vi "Read Variant Key.vi"(5 "format string (%;%f)":string="%f", 7 "section":string, 8 "error in (no error)":errorcluster, 9 "type":variant, 10 "key (optional)":string, 11 "refnum":T1) -> (0 "error out":errorcluster, 1 "key-value":variant, 2 "found?":bool, 3 "refnum out":T1)   [LabVIEW 2017, in "INI++.lvlib"]
doc: "Reads a value associated with key in a specified section of the configuration data identified by refnum. If \"key\" input is not specified, the name of the variant object is used as the key. the \"found?\" output will be TRUE for compount objects (clusters) only if all elements (recursively) are found.\n\nFor example a Boolean named \"Enable\" with a value of TRUE would correspond to the key-value pair:\n\nEnable=TRUE\n\nNote: Special characters in section and key names will be escape-coded. These include the following: \\00-\\1F (non-printable chars); \"[\", \"]\", and \"=\" (INI syntax elements); \\FE (\"þ\") and \\FF (\"ÿ\") (legacy bracket encoding); Additionally, the escape character, \"\\\", will be escaped as \"\\\\\"."
uses:
  Candidate/INI/INI++.lvlib
  <vilib>/Utility/config.llb/NI_LVConfig.lvlib
  <vilib>/Utility/config.llb/Read Key (String).vi
  <vilib>/Utility/config.llb/Read Key (Double).vi
  <vilib>/Utility/Data Type/NI_Data Type.lvlib
  <vilib>/Utility/Data Type/Type Definitions/Data Type.ctl
  _openG/_reuse_openG.lvlib
  <vilib>/Utility/config.llb/Read Key (Boolean).vi
  <vilib>/Utility/config.llb/Read Key (Path).vi
  <vilib>/Utility/config.llb/Read Key (U32).vi
  <vilib>/Utility/config.llb/Read Key (I32).vi
  <vilib>/Utility/config.llb/Config Data RefNum.ctl
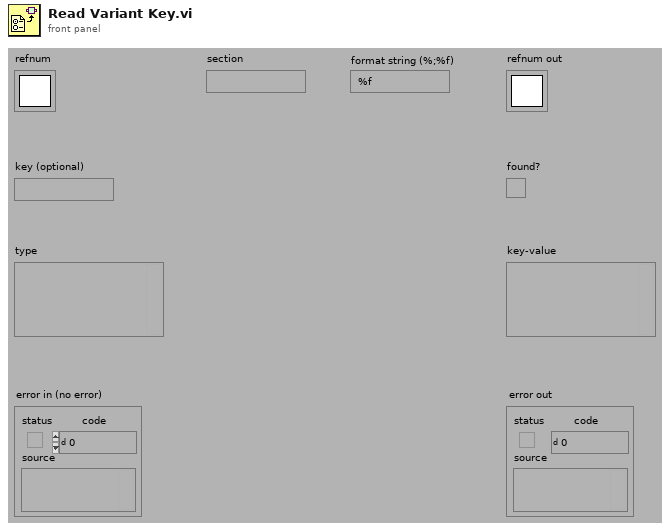
[diagram p1: front panel]
types:
  T1 = typedef "NI_LVConfig.lvlib/Config Data RefNum.ctl" = refnum<k1>
  T2 = typedef "NI_Data Type.lvlib/Data Type.ctl" = enum8{"Invalid Type", "Void", "I8", "I16", "I32", "I64", "U8", "U16", "U32", "U64", "Single Float", "Double Float", "Extended Float", "Single Complex", "Double Complex", "Extended Complex", "Enum U8", "Enum U16", "Enum U32", "Enum U64", "Single Float With Unit", "Double Float With Unit", "Extended Float With Unit", "Single Complex with Unit", "Double Complex with Unit", "Extended Complex with Unit", "Boolean", "String", "Path", "Picture", "Tag", "Array", "Cluster", "Variant", "LV Variant", "Waveform", "Timestamp", "Digital Waveform", "Digital Data", "ExpressData", "Refnum", "External Data", "VI", "Poly VI", "LabVIEW Class Instance", "Fixed Point"}
  T3 = typedef "Type Descriptor__ogtk.ctl" = i16[]
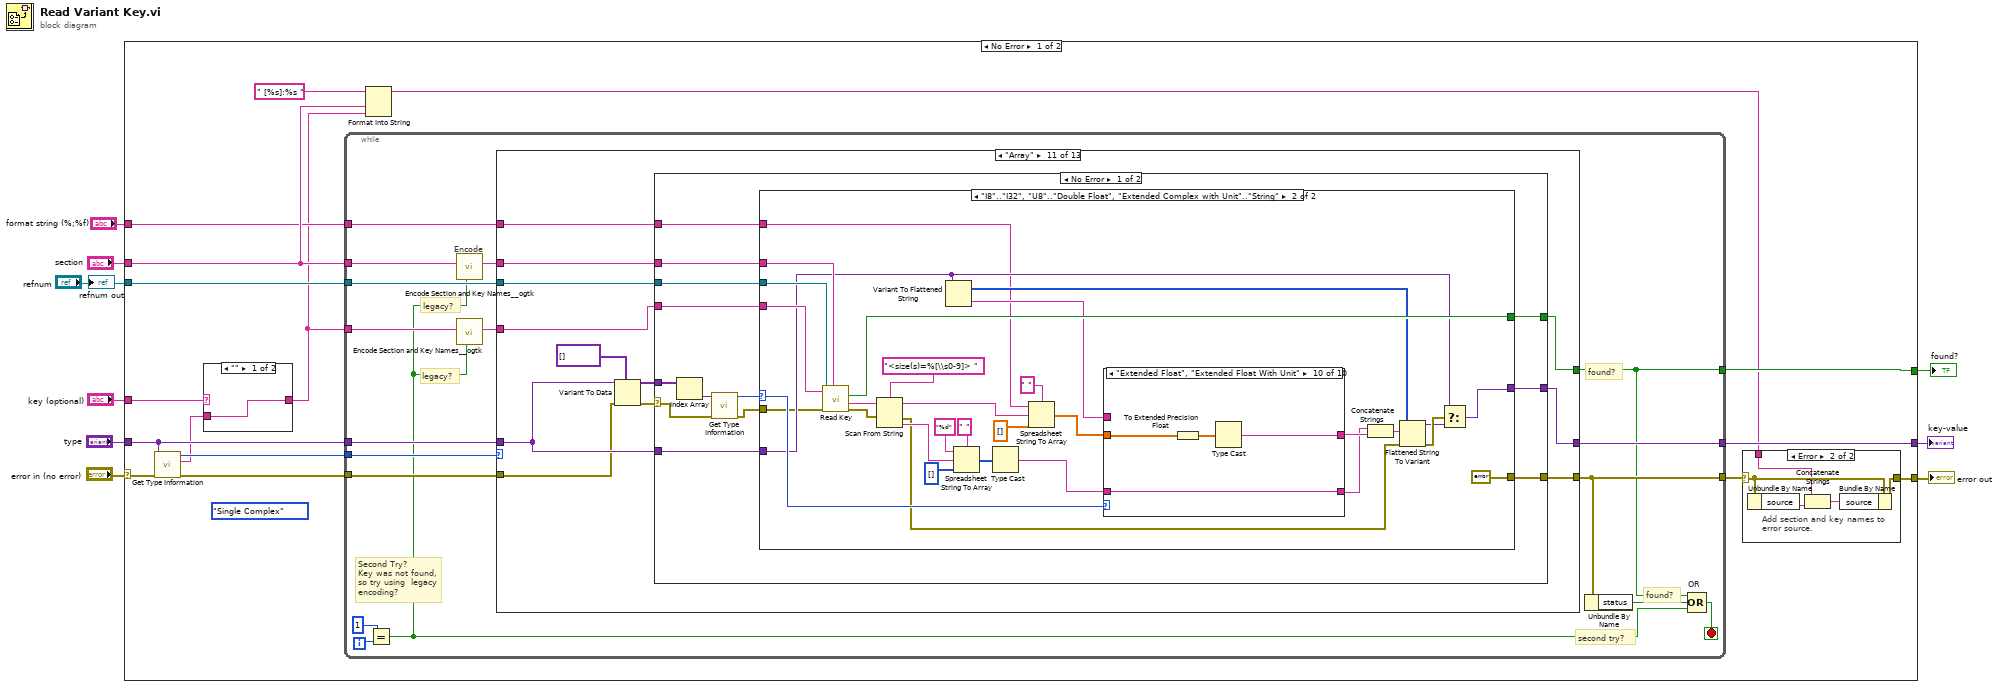
[diagram p0: block diagram]
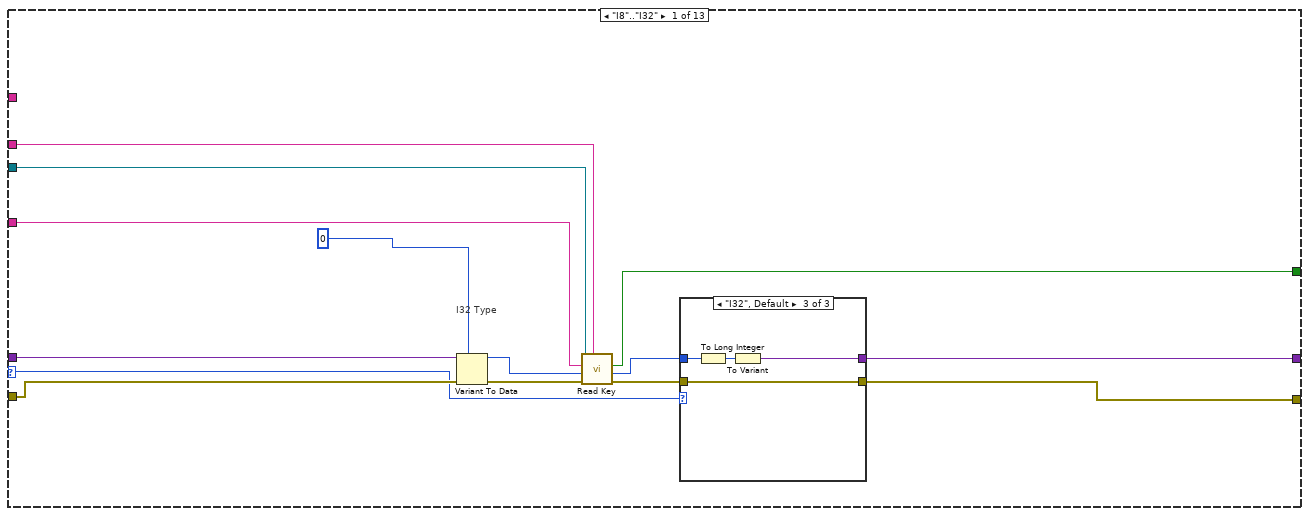
[diagram p3: hidden frame]
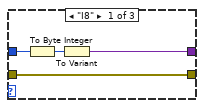
[diagram p4: hidden frame]
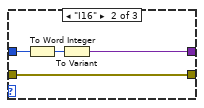
[diagram p5: hidden frame]
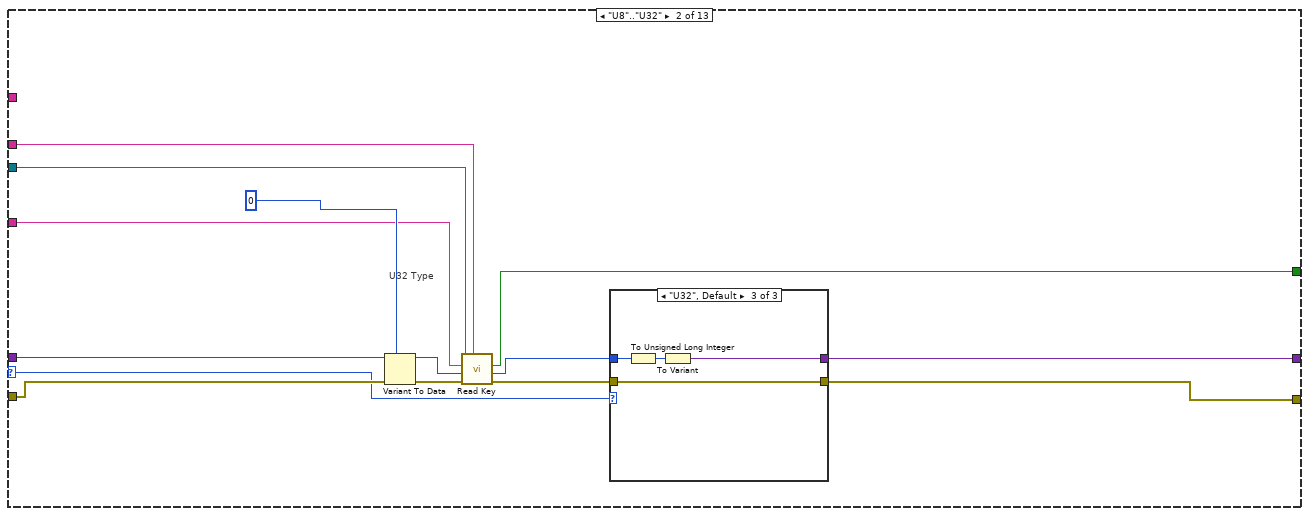
[diagram p6: hidden frame]
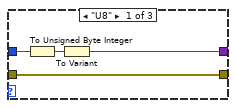
[diagram p7: hidden frame]
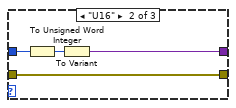
[diagram p8: hidden frame]
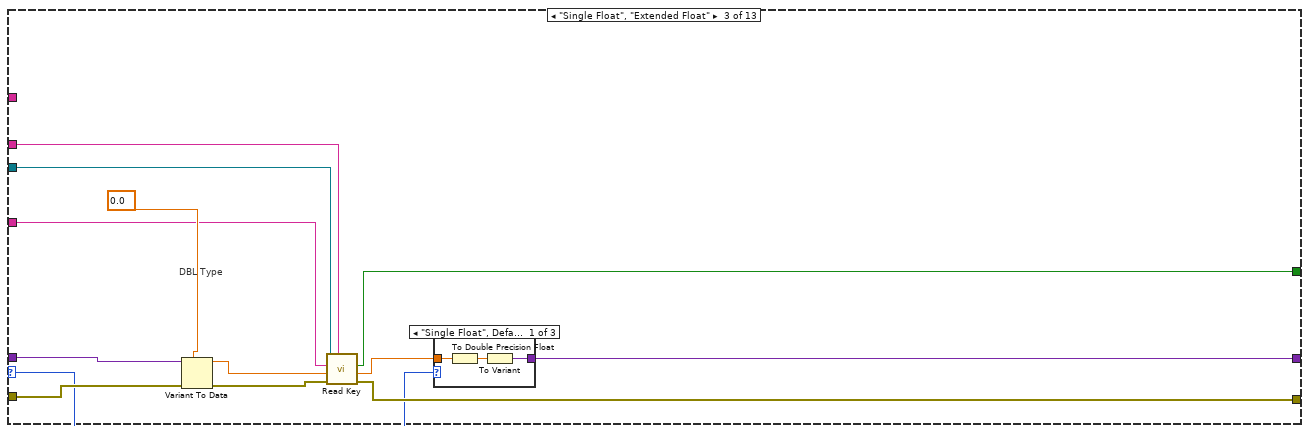
[diagram p9: hidden frame]
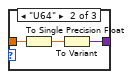
[diagram p10: hidden frame]
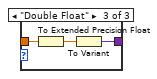
[diagram p11: hidden frame]
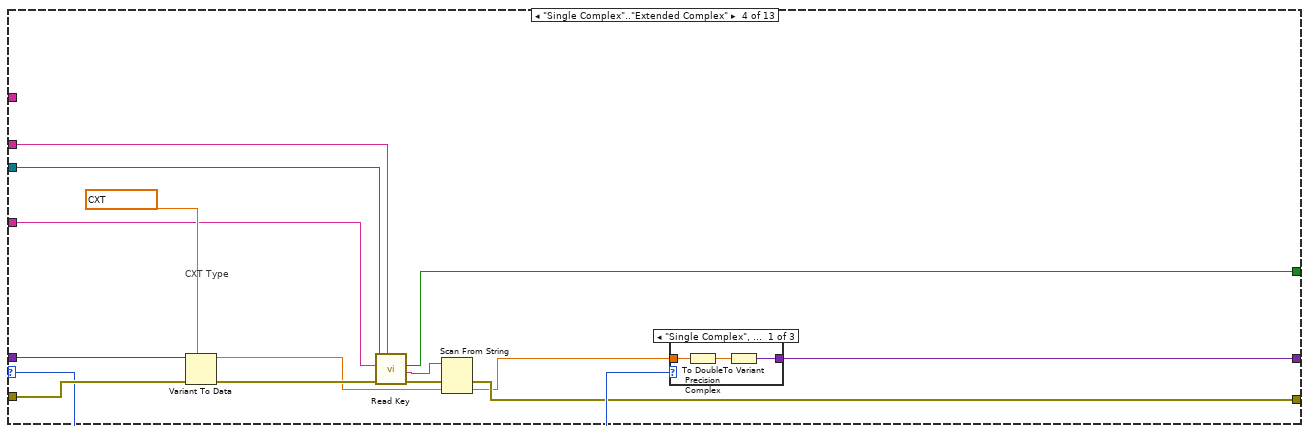
[diagram p12: hidden frame]
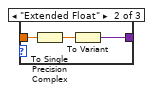
[diagram p13: hidden frame]
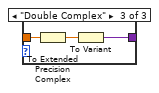
[diagram p14: hidden frame]
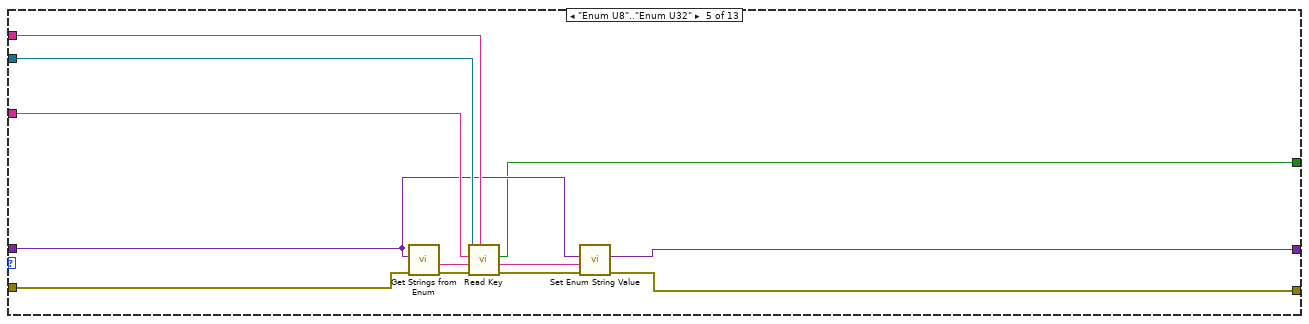
[diagram p15: hidden frame]
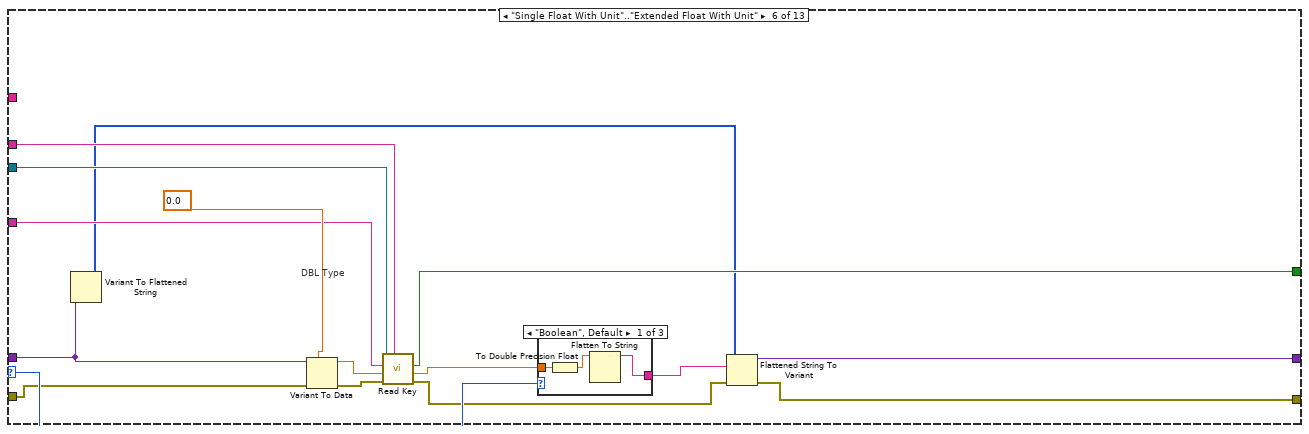
[diagram p16: hidden frame]
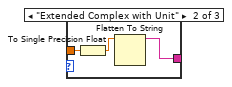
[diagram p17: hidden frame]
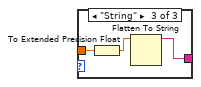
[diagram p18: hidden frame]
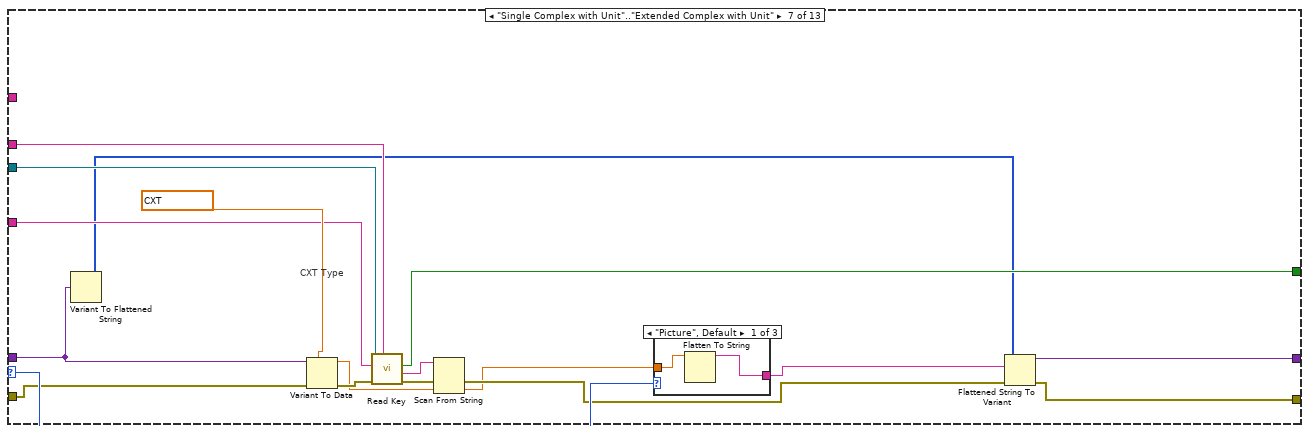
[diagram p19: hidden frame]
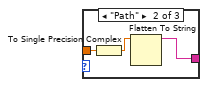
[diagram p20: hidden frame]
diagram:
  n1 = case shown="No Error" "error in (no error)" {
    selector: "error in (no error)" -> [w23 w454]
    tunnel: "refnum" -> [w25 _]
    tunnel: [w18 w454] -> w9
    tunnel: "type" -> [w21 _]
    tunnel: "key (optional)" -> [w12 _]
    tunnel: "section" -> [w15 _]
    tunnel: [w24 variant ("Variant")] -> w4
    tunnel: [w20 FALSE ("found?")] -> w2
    tunnel: "format string (%;%f)" -> [w14 _]
    frame No Error {
      (unwired) Data_Type."Single Complex" ("Type")
      n2 = call <vilib>:"Get Type Information.vi"("error in (no error)"=w23, "Variant"=w21) -> ("error out"=w22:errorcluster, "Name"=w10:string, "Type"=w13:T2)  [unwired: 5 in, 2 out]
      n3 = case shown="\"\"" w12 {
        selector: w12 -> [_ w27]
        tunnel: [w26 w27] -> w11
        tunnel: w10 -> [w26 _]
        frame "" {
        }
        frame Default {
        }
      }
      n4 = while {
        tunnel: w13 -> [w44]
        tunnel: w25 -> [w43]
        tunnel: [w42] -> w24
        tunnel: w22 -> [w41]
        tunnel: w21 -> [w40]
        tunnel: [w33] -> w20
        tunnel: [w35] -> w19
        tunnel: w15 -> [w38]
        tunnel: w11 -> [w37]
        tunnel: w14 -> [w28]
        i -> [w32]
        stop <- w30 stop-if-true
        # "found?"
        # "found?"
        # "second try?"
        # "legacy?"
        # "legacy?"
        # "Second Try?\nKey was not found, so try using  legacy encoding?"
        # "Encode"
        n5 = Equal?(x=1, y=w32) -> (x = y?=w29:bool)
        n6 = call <userlib>:"Encode Section and Key Names__ogtk.vi"("use legacy encoding scheme? (FALSE)"=w29, "string"=w38) -> ("encoded string"=w39:string)  [unwired: 9 in]
        n7 = call <userlib>:"Encode Section and Key Names__ogtk.vi"("use legacy encoding scheme? (FALSE)"=w29, "string"=w37) -> ("encoded string"=w36:string)  [unwired: 9 in]
        n8 = case shown="\"Array\"" w44 {
          selector: w44 -> [w47 w73 w97 w124 _ w162 w191 _ _ _ _ _ _]
          tunnel: w40 -> [w57 w83 w108 w132 w145 w157 w187 w216 w228 w240 w246 w402 w442]
          tunnel: w43 -> [w56 w82 w107 w131 w154 w169 w196 w215 w227 w239 w253 w407 w445]
          tunnel: [w46 w71 w105 w122 w147 w159 w189 w213 w225 w237 w251 w405 w436] -> w35
          tunnel: w41 -> [w54 w80 w104 w129 w151 w161 w190 w212 w224 w236 w242 w406 w438]
          tunnel: w36 -> [w53 w79 w103 w128 w153 w167 w194 w211 w223 w235 w248 w408 w444]
          tunnel: w39 -> [w52 w78 w102 w127 w152 w166 w193 w210 w222 w234 w249 w409 w443]
          tunnel: [w45 w75 w99 w126 w144 w155 w185 w207 w221 w231 w252 w404 w439] -> w42
          tunnel: [w50 w74 w98 w125 w143 w163 w192 w206 w218 w230 w250 w403 w434] -> w33
          tunnel: w28 -> [_ _ _ _ _ _ _ _ _ _ w247 w410 _]
          frame "I8".."I32" {
            # "I32 Type"
            n9 = Variant To Data(error in=w54, type=0, Variant=w57) -> (data=w51:i32, error out=w55:errorcluster)
            n10 = call-poly <vilib>:"Read Key.vi"("section"=w52, "error in (no error)"=w55, "default value"=w51, "key"=w53, "refnum"=w56) -> ("error out"=w49:errorcluster, "value"=w48:i32, "found?"=w50:bool)  [unwired: 3 in, 1 out]
            n11 = case shown="\"I32\", Default" w47 {
              tunnel: w48 -> [w62 w66 w70]
              tunnel: [w61 w65 w69] -> w45
              tunnel: w49 -> [w59 w63 w67]
              tunnel: [w59 w63 w67] -> w46
              frame "I8" {
                n12 = To Byte Integer(number=w62) -> (8bit integer=w60:i8)
                n13 = To Variant(anything=w60) -> (Variant=w61:variant)
              }
              frame "I16" {
                n14 = To Word Integer(number=w66) -> (16bit integer=w64:i16)
                n15 = To Variant(anything=w64) -> (Variant=w65:variant)
              }
              frame "I32", Default {
                n16 = To Long Integer(number=w70) -> (32bit integer=w68:i32)
                n17 = To Variant(anything=w68) -> (Variant=w69:variant)
              }
            }
          }
          frame "U8".."U32" {
            # "U32 Type"
            n18 = Variant To Data(error in=w80, type=u32 0, Variant=w83) -> (data=w77:u32, error out=w81:errorcluster)
            n19 = call-poly <vilib>:"Read Key.vi"("section"=w78, "error in (no error)"=w81, "default value"=w77, "key"=w79, "refnum"=w82) -> ("error out"=w72:errorcluster, "value"=w76:u32, "found?"=w74:bool)  [unwired: 3 in, 1 out]
            n20 = case shown="\"U32\", Default" w73 {
              tunnel: w76 -> [w88 w92 w96]
              tunnel: [w87 w91 w95] -> w75
              tunnel: w72 -> [w85 w89 w93]
              tunnel: [w85 w89 w93] -> w71
              frame "U8" {
                n21 = To Unsigned Byte Integer(number=w88) -> (unsigned 8bit integer=w86:u8)
                n22 = To Variant(anything=w86) -> (Variant=w87:variant)
              }
              frame "U16" {
                n23 = To Unsigned Word Integer(number=w92) -> (unsigned 16bit integer=w90:u16)
                n24 = To Variant(anything=w90) -> (Variant=w91:variant)
              }
              frame "U32", Default {
                n25 = To Unsigned Long Integer(number=w96) -> (unsigned 32bit integer=w94:u32)
                n26 = To Variant(anything=w94) -> (Variant=w95:variant)
              }
            }
          }
          frame "Single Float", "Extended Float" {
            # "DBL Type"
            n27 = Variant To Data(error in=w104, type=0.0, Variant=w108) -> (data=w101:dbl, error out=w106:errorcluster)
            n28 = call-poly <vilib>:"Read Key.vi"("section"=w102, "error in (no error)"=w106, "default value"=w101, "key"=w103, "refnum"=w107) -> ("error out"=w105:errorcluster, "value"=w100:dbl, "found?"=w98:bool)  [unwired: 3 in, 1 out]
            n29 = case shown="\"Single Float\", Default" w97 {
              tunnel: w100 -> [w112 w115 w118]
              tunnel: [w111 w114 w117] -> w99
              frame "Single Float", Default {
                n30 = To Double Precision Float(number=w112) -> (double precision float=w110:dbl)
                n31 = To Variant(anything=w110) -> (Variant=w111:variant)
              }
              frame "U64" {
                n32 = To Single Precision Float(number=w115) -> (single precision float=w113:sgl)
                n33 = To Variant(anything=w113) -> (Variant=w114:variant)
              }
              frame "Double Float" {
                n34 = To Extended Precision Float(1:w118) -> (0:w116:ext)
                n35 = To Variant(anything=w116) -> (Variant=w117:variant)
              }
            }
          }
          frame "Single Complex".."Extended Complex" {
            # "CXT Type"
            n36 = Variant To Data(error in=w129, type=cxt 0.0+0.0i, Variant=w132) -> (data=w120:cxt, error out=w130:errorcluster)
            n37 = call-poly <vilib>:"Read Key.vi"("section"=w127, "error in (no error)"=w130, "key"=w128, "refnum"=w131) -> ("error out"=w123:errorcluster, "value"=w121:string, "found?"=w125:bool)  [unwired: 4 in, 1 out]
            n38 = Scan From String(input string=w121, error in=w123, default 1=w120) -> (error out=w122:errorcluster, output 1=w119:cxt)  [unwired: 2 in, 2 out]
            n39 = case shown="\"Single Complex\", Default" w124 {
              tunnel: w119 -> [w136 w139 w142]
              tunnel: [w135 w138 w141] -> w126
              frame "Single Complex", Default {
                n40 = To Double Precision Complex(1:w136) -> (0:w134:cdb)
                n41 = To Variant(anything=w134) -> (Variant=w135:variant)
              }
              frame "Extended Float" {
                n42 = To Single Precision Complex(1:w139) -> (0:w137:csg)
                n43 = To Variant(anything=w137) -> (Variant=w138:variant)
              }
              frame "Double Complex" {
                n44 = To Extended Precision Complex(1:w142) -> (0:w140:cxt)
                n45 = To Variant(anything=w140) -> (Variant=w141:variant)
              }
            }
          }
          frame "Enum U8".."Enum U32" {
            n46 = call "Get Strings from Enum.vi"("error in (no error)"=w151, "Enum"=w145) -> ("error out"=w150:errorcluster, "String Value"=w149:string)  [unwired: 6 in, 2 out]
            n47 = call-poly <vilib>:"Read Key.vi"("section"=w152, "error in (no error)"=w150, "default value"=w149, "key"=w153, "refnum"=w154) -> ("error out"=w148:errorcluster, "value"=w146:string, "found?"=w143:bool)  [unwired: 3 in, 1 out]
            n48 = call "Set Enum String Value.vi"("error in (no error)"=w148, "String Value"=w146, "Default Enum Value"=w145) -> ("error out"=w147:errorcluster, "Enum"=w144:variant)  [unwired: 7 in]
          }
          frame "Single Float With Unit".."Extended Float With Unit" {
            # "DBL Type"
            n49 = Variant To Flattened String(Variant=w157) -> (1:w156:i16[])  [unwired: 1 out]
            n50 = Variant To Data(error in=w161, type=0.0, Variant=w157) -> (data=w165:dbl, error out=w168:errorcluster)
            n51 = call-poly <vilib>:"Read Key.vi"("section"=w166, "error in (no error)"=w168, "default value"=w165, "key"=w167, "refnum"=w169) -> ("error out"=w160:errorcluster, "value"=w164:dbl, "found?"=w163:bool)  [unwired: 3 in, 1 out]
            n52 = case shown="\"Boolean\", Default" w162 {
              tunnel: w164 -> [w173 w176 w179]
              tunnel: [w172 w174 w177] -> w158
              frame "Boolean", Default {
                n53 = To Double Precision Float(number=w173) -> (double precision float=w171:dbl)
                n54 = Flatten To String(anything=w171) -> (data string=w172:string)  [unwired: 3 in, 2 out]
              }
              frame "Extended Complex with Unit" {
                n55 = To Single Precision Float(number=w176) -> (single precision float=w175:sgl)
                n56 = Flatten To String(anything=w175) -> (data string=w174:string)  [unwired: 3 in, 2 out]
              }
              frame "String" {
                n57 = To Extended Precision Float(1:w179) -> (0:w178:ext)
                n58 = Flatten To String(anything=w178) -> (data string=w177:string)  [unwired: 3 in, 2 out]
              }
            }
            n59 = Flattened String To Variant(4:w160, 6:w158, 7:w156) -> (0:w159:errorcluster, 3:w155:variant)
          }
          frame "Single Complex with Unit".."Extended Complex with Unit" {
            # "CXT Type"
            n60 = Variant To Flattened String(Variant=w187) -> (1:w186:i16[])  [unwired: 1 out]
            n61 = Variant To Data(error in=w190, type=cxt 0.0+0.0i, Variant=w187) -> (data=w181:cxt, error out=w195:errorcluster)
            n62 = call-poly <vilib>:"Read Key.vi"("section"=w193, "error in (no error)"=w195, "key"=w194, "refnum"=w196) -> ("error out"=w183:errorcluster, "value"=w182:string, "found?"=w192:bool)  [unwired: 4 in, 1 out]
            n63 = Scan From String(input string=w182, error in=w183, default 1=w181) -> (error out=w184:errorcluster, output 1=w180:cxt)  [unwired: 2 in, 2 out]
            n64 = case shown="\"Picture\", Default" w191 {
              tunnel: w180 -> [w199 w202 w205]
              tunnel: [w198 w200 w203] -> w188
              frame "Picture", Default {
                n65 = Flatten To String(anything=w199) -> (data string=w198:string)  [unwired: 3 in, 2 out]
              }
              frame "Path" {
                n66 = To Single Precision Complex(1:w202) -> (0:w201:csg)
                n67 = Flatten To String(anything=w201) -> (data string=w200:string)  [unwired: 3 in, 2 out]
              }
              frame "Tag" {
                n68 = To Extended Precision Complex(1:w205) -> (0:w204:cxt)
                n69 = Flatten To String(anything=w204) -> (data string=w203:string)  [unwired: 3 in, 2 out]
              }
            }
            n70 = Flattened String To Variant(4:w184, 6:w188, 7:w186) -> (0:w189:errorcluster, 3:w185:variant)
          }
          frame "Boolean" {
            # "Boolean Type"
            n71 = Variant To Data(error in=w212, type=FALSE, Variant=w216) -> (data=w209:bool, error out=w214:errorcluster)
            n72 = call-poly <vilib>:"Read Key.vi"("section"=w210, "error in (no error)"=w214, "default value"=w209, "key"=w211, "refnum"=w215) -> ("error out"=w213:errorcluster, "value"=w208:bool, "found?"=w206:bool)  [unwired: 3 in, 1 out]
            n73 = To Variant(anything=w208) -> (Variant=w207:variant)
          }
          frame "String", "Tag" {
            # "String Type"
            n74 = Variant To Data(error in=w224, type="", Variant=w228) -> (data=w219:string, error out=w226:errorcluster)
            n75 = call-poly <vilib>:"Read Key.vi"("section"=w222, "error in (no error)"=w226, "default value"=w219, "key"=w223, "refnum"=w227) -> ("error out"=w225:errorcluster, "value"=w220:string, "found?"=w218:bool)  [unwired: 3 in, 1 out]
            n76 = To Variant(anything=w220) -> (Variant=w221:variant)
          }
          frame "Path" {
            # "Path Type"
            n77 = Variant To Data(error in=w236, type=path "", Variant=w240) -> (data=w233:path, error out=w238:errorcluster)
            n78 = call-poly <vilib>:"Read Key.vi"("section"=w234, "error in (no error)"=w238, "default value"=w233, "key"=w235, "refnum"=w239) -> ("error out"=w237:errorcluster, "value"=w232:path, "found?"=w230:bool)  [unwired: 3 in, 1 out]
            n79 = To Variant(anything=w232) -> (Variant=w231:variant)
          }
          frame "Array" {
            n80 = Variant To Data(error in=w242, type=variant[] [], Variant=w246) -> (data=w244:variant[], error out=w243:errorcluster)
            n81 = case shown="No Error" w243 {
              selector: w243 -> [w254 _]
              tunnel: w253 -> [w266 w394]
              tunnel: [w265 w390] -> w252
              tunnel: [w264 w391] -> w251
              tunnel: [w263 _] -> w250
              tunnel: w249 -> [w262 w392]
              tunnel: w248 -> [w261 w393]
              tunnel: w247 -> [w260 _]
              tunnel: w246 -> [w259 w395]
              tunnel: w244 -> [w258 _]
              frame No Error {
                n82 = Index Array(array=w258) -> (element=w257:variant)  [unwired: 1 in]
                n83 = call <vilib>:"Get Type Information.vi"("error in (no error)"=w254, "Variant"=w257) -> ("error out"=w255:errorcluster, "Type"=w256:T2)  [unwired: 5 in, 3 out]
                n84 = case shown="\"I8\"..\"I32\", \"U8\"..\"Double Float\", \"Extended Complex with Unit\"..\"String\"" w256 {
                  selector: w256 -> [_ w337]
                  tunnel: w255 -> [w267 w321]
                  tunnel: w259 -> [w276 w325]
                  tunnel: w262 -> [w275 w347]
                  tunnel: w266 -> [w274 w348]
                  tunnel: w261 -> [w277 w349]
                  tunnel: [w272 w324] -> w265
                  tunnel: [w271 errorcluster {"status"=FALSE, "code"=0, "source"=""} ("error out")] -> w264
                  tunnel: [w270 w346] -> w263
                  tunnel: w260 -> [w268 w322]
                  frame Default {
                    n85 = Concatenate Strings(w277, ".<size(s)>" ("Substring")) -> (w280:string)
                    n86 = call-poly <vilib>:"Read Key.vi"("read raw string? (F)"=TRUE, "section"=w275, "error in (no error)"=w267, "key"=w280, "refnum"=w274) -> ("error out"=w278:errorcluster, "value"=w279:string, "found?"=w269:bool)  [unwired: 3 in, 1 out]
                    n87 = case shown="True" w269 {
                      tunnel: w279 -> [_ w306]
                      tunnel: w278 -> [_ w287]
                      tunnel: w277 -> [_ w303]
                      tunnel: w276 -> [w283 w302]
                      tunnel: w275 -> [_ w301]
                      tunnel: w274 -> [_ w300]
                      tunnel: [w283 w294] -> w272
                      tunnel: [errorcluster {"status"=FALSE, "code"=0, "source"=""} ("error out") w293] -> w271
                      tunnel: [FALSE w291] -> w270
                      tunnel: w268 -> [_ w286]
                      frame False {
                        # "array size(s) not found. Ignore element keys (if any) and return input array"
                      }
                      frame True {
                        # "array.size(s) is found. Read elements keys. missing keys replace with datatype default."
                        n88 = call <userlib>:"Get Array Element TD__ogtk.vi"("error in (no error)"=w287, "Array"=w302) -> ("error out"=w289:errorcluster, "Type Descriptor"=w290:T3)  [unwired: 8 in]
                        n89 = call <userlib>:"Get Default Data from TD__ogtk.vi"("error in (no error)"=w289, "Type Descriptor"=w290) -> ("error out"=w285:errorcluster, "Default VData"=w288:variant)  [unwired: 8 in]
                        n90 = Spreadsheet String To Array(delimiter (Tab)=" ", format string="%d", spreadsheet string=w306, array type (2D Dbl)=u32[] [] ("Array Constant")) -> (array=w295:u32[])
                        n91 = Multiply Array Elements(1:w295) -> (0:w304:u32)
                        n92 = for {
                          N: w304 -> [_]
                          shift-right: [w311] -> w298
                          shift-left: w285 -> [w312]
                          tunnel: w303 -> [w318]
                          tunnel: w288 -> [w317]
                          tunnel: w301 -> [w310]
                          tunnel: w300 -> [w315]
                          tunnel: [w314] -> w299 mode=indexing
                          tunnel: [w313] -> w292 mode=indexing
                          tunnel: w286 -> [w309]
                          i -> [w319]
                          n93 = Format Into String(format string=" %d" ("Format String"), initial string=w318, w319) -> (resulting string=w316:string)  [unwired: 1 in, 1 out]
                          n94 = call "Read Variant Key.vi"("format string (%;%f)"=w309, "section"=w310, "error in (no error)"=w312, "type"=w317, "key (optional)"=w316, "refnum"=w315) -> ("error out"=w311:errorcluster, "key-value"=w314:variant, "found?"=w313:bool)  [unwired: 2 in, 1 out]
                        }
                        n95 = And Array Elements(Boolean array=w292) -> (logical AND=w291:bool)
                        n96 = call <userlib>:"Array of VData to VArray__ogtk.vi"("error in (no error)"=w298, "Element Type (when empty)"=w288, "1D Array of VData"=w299) -> ("error out"=w297:errorcluster, "VArray"=w296:variant)  [unwired: 7 in]
                        n97 = call <userlib>:"Reshape 1D Array__ogtk.vi"("error in (no error)"=w297, "Size(s)"=w295, "1D Array"=w296) -> ("error out"=w293:errorcluster, "Reshaped VArray"=w294:variant)  [unwired: 7 in]
                      }
                    }
                  }
                  frame "I8".."I32", "U8".."Double Float", "Extended Complex with Unit".."String" {
                    n98 = call-poly <vilib>:"Read Key.vi"("section"=w347, "error in (no error)"=w321, "key"=w349, "refnum"=w348) -> ("error out"=w345:errorcluster, "value"=w350:string, "found?"=w346:bool)  [unwired: 4 in, 1 out]
                    n99 = Scan From String(format string="<size(s)=%[\\s0-9]> " ("regular expression"), input string=w350, error in=w345) -> (remaining string=w338:string, error out=w328:errorcluster, output 1=w343:string)  [unwired: 2 in, 1 out]
                    n100 = Variant To Flattened String(Variant=w325) -> (data string=w330:string, 1:w331:i16[])
                    n101 = Spreadsheet String To Array(delimiter (Tab)=" ", format string="%d", spreadsheet string=w343, array type (2D Dbl)=u32[] []) -> (array=w344:u32[])
                    n102 = Type Cast(x=w344) -> (*(type *) &x=w335:string)  [unwired: 1 in]
                    n103 = Spreadsheet String To Array(delimiter (Tab)=" ", format string=w322, spreadsheet string=w338, array type (2D Dbl)=dbl[] []) -> (array=w336:dbl[])
                    n104 = case shown="\"Extended Float\", \"Extended Float With Unit\"" w337 {
                      tunnel: w336 -> [_ w357 w361 w365 w369 w373 w377 w381 w383 w387]
                      tunnel: [w352 w355 w359 w363 w367 w371 w375 w379 w385 w389] -> w333
                      tunnel: ["" w354 w358 w362 w366 w370 w374 w378 w384 w388] -> w332
                      tunnel: w335 -> [_ w354 w358 w362 w366 w370 w374 w378 w384 w388]
                      tunnel: w330 -> [w352 _ _ _ _ _ _ _ _ _]
                      frame Default {
                      }
                      frame "I8" {
                        n105 = To Byte Integer(number=w357) -> (8bit integer=w356:i8[])
                        n106 = Type Cast(x=w356) -> (*(type *) &x=w355:string)  [unwired: 1 in]
                      }
                      frame "I16" {
                        n107 = To Word Integer(number=w361) -> (16bit integer=w360:i16[])
                        n108 = Type Cast(x=w360) -> (*(type *) &x=w359:string)  [unwired: 1 in]
                      }
                      frame "I32" {
                        n109 = To Long Integer(number=w365) -> (32bit integer=w364:i32[])
                        n110 = Type Cast(x=w364) -> (*(type *) &x=w363:string)  [unwired: 1 in]
                      }
                      frame "U8" {
                        n111 = To Unsigned Byte Integer(number=w369) -> (unsigned 8bit integer=w368:u8[])
                        n112 = Type Cast(x=w368) -> (*(type *) &x=w367:string)  [unwired: 1 in]
                      }
                      frame "U16" {
                        n113 = To Unsigned Word Integer(number=w373) -> (unsigned 16bit integer=w372:u16[])
                        n114 = Type Cast(x=w372) -> (*(type *) &x=w371:string)  [unwired: 1 in]
                      }
                      frame "U32" {
                        n115 = To Unsigned Long Integer(number=w377) -> (unsigned 32bit integer=w376:u32[])
                        n116 = Type Cast(x=w376) -> (*(type *) &x=w375:string)  [unwired: 1 in]
                      }
                      frame "Single Float", "Single Float With Unit" {
                        n117 = To Single Precision Float(number=w381) -> (single precision float=w380:sgl[])
                        n118 = Type Cast(x=w380) -> (*(type *) &x=w379:string)  [unwired: 1 in]
                      }
                      frame "Double Float", "Double Float With Unit" {
                        n119 = To Double Precision Float(number=w383) -> (double precision float=w382:dbl[])
                        n120 = Type Cast(x=w382) -> (*(type *) &x=w385:string)  [unwired: 1 in]
                      }
                      frame "Extended Float", "Extended Float With Unit" {
                        n121 = To Extended Precision Float(1:w387) -> (0:w386:ext[])
                        n122 = Type Cast(x=w386) -> (*(type *) &x=w389:string)  [unwired: 1 in]
                      }
                    }
                    n123 = Concatenate Strings(w332, w333) -> (w334:string)
                    n124 = Flattened String To Variant(4:w328, 6:w334, 7:w331) -> (0:w327:errorcluster, 3:w326:variant)
                    n125 = Select(t=w325, s=w327, f=w326) -> (s? t:f=w324:variant)
                  }
                }
              }
              frame Error {
                n126 = Variant To Flattened String(Variant=w395) -> (data string=w400:string, 1:w397:i16[])
                n127 = call-poly <vilib>:"Read Key.vi"("section"=w392, "default value"=w400, "key"=w393, "refnum"=w394) -> ("error out"=w398:errorcluster, "value"=w399:string, "found?"=w396:bool)  [unwired: 4 in, 1 out]
                n128 = Flattened String To Variant(4:w398, 6:w399, 7:w397) -> (0:w391:errorcluster, 3:w390:variant)
              }
            }
          }
          frame "Cluster" {
            # ">> Cluster Name >>"
            # "Expand cluster to its elements\nand read keys recursively."
            n129 = call <vilib>:"Get Type Information.vi"("error in (no error)"=w406, "Variant"=w402) -> ("error out"=w412:errorcluster, "Name"=w411:string)  [unwired: 5 in, 3 out]
            n130 = call "ClusterToArray.vi"("Error in"=w412, "Cluster"=w402) -> ("Error out"=w401:errorcluster, "Array"=w418:variant[])  [unwired: 8 in]
            n131 = for {
              shift-right: [w426] -> w416
              shift-left: w401 -> [w431]
              tunnel: w418 -> [w423] mode=indexing
              tunnel: w409 -> [w420]
              tunnel: w407 -> [w429]
              tunnel: w408 -> [w433]
              tunnel: [w427] -> w417 mode=indexing
              tunnel: [w424] -> w415 mode=indexing
              tunnel: w410 -> [w419]
              n132 = call <vilib>:"Get Type Information.vi"("error in (no error)"=w431, "Variant"=w423) -> ("error out"=w422:errorcluster, "Name"=w425:string)  [unwired: 5 in, 3 out]
              n133 = Format Into String(format string=".%s" ("Format String"), initial string=w433, w425) -> (resulting string=w430:string)  [unwired: 1 in, 1 out]
              n134 = call "Read Variant Key.vi"("format string (%;%f)"=w419, "section"=w420, "error in (no error)"=w422, "type"=w423, "key (optional)"=w430, "refnum"=w429) -> ("error out"=w421:errorcluster, "key-value"=w428:variant, "found?"=w424:bool)  [unwired: 2 in, 1 out]
              n135 = call "Set Data Name.vi"("error in (no error)"=w421, "Data Name"=w425, "Data"=w428) -> ("error out"=w426:errorcluster, "Renamed Data"=w427:variant)  [unwired: 7 in]
            }
            n136 = And Array Elements(Boolean array=w415) -> (logical AND=w403:bool)
            n137 = call "ArrayToCluster.vi"("Error in"=w416, "Array"=w417) -> ("Error out"=w414:errorcluster, "Cluster"=w413:variant)  [unwired: 8 in]
            n138 = call "Set Data Name.vi"("error in (no error)"=w414, "Data Name"=w411, "Data"=w413) -> ("error out"=w405:errorcluster, "Renamed Data"=w404:variant)  [unwired: 7 in]
          }
          frame Default {
            n139 = Variant To Flattened String(Variant=w442) -> (data string=w441:string, 1:w435:i16[])
            n140 = call-poly <vilib>:"Read Key.vi"("section"=w443, "error in (no error)"=w438, "default value"=w441, "key"=w444, "refnum"=w445) -> ("error out"=w437:errorcluster, "value"=w440:string, "found?"=w434:bool)  [unwired: 3 in, 1 out]
            n141 = Flattened String To Variant(4:w437, 6:w440, 7:w435) -> (0:w436:errorcluster, 3:w439:variant)
          }
        }
        n142 = Unbundle By Name(w35) -> ("status"=w34:bool)
        n143 = Compound Arithmetic op=OR "OR"(w33, w34, w29) -> (w30:bool)
      }
      n144 = Format Into String(format string=" [%s]:%s " ("Format String"), w15, w11) -> (resulting string=w16:string)  [unwired: 2 in, 1 out]
      n145 = case shown="Error" w19 {
        selector: w19 -> [w446 w451]
        tunnel: [w446 w450] -> w18
        tunnel: w16 -> [_ w447]
        frame No Error {
        }
        frame Error {
          # "Add section and key names to\nerror source."
          n146 = Unbundle By Name(w451) -> ("source"=w448:string)
          n147 = Concatenate Strings(w447, w448) -> (w449:string)
          n148 = Bundle By Name(cluster=w451, "source"=w449) -> (w450:errorcluster)
        }
      }
    }
    frame Error {
    }
  }
  "error out" <- w9
  "key-value" <- w4
  "found?" <- w2
  "refnum out" <- "refnum"
